vi "PC Streaming Host with slow - original.vi"() -> ()   [LabVIEW 2012]
uses:
  <vilib>/userdefined/High Color/nirio_resource_hc.ctl
  hv cluster control.ctl
  Slow cluster control.ctl
  <vilib>/FPGAPlugInAG/PXI-7951R/niLvFpga_Open_PXI-7951R.vi
  <vilib>/rvi/interface/common/dynamic/niFpgaDynamicAddResources.vi
  <vilib>/Utility/error.llb/Error Cluster From Error Code.vi
  <vilib>/rvi/errors/niLvFpgaAdjustHostInterfaceError.vi
  <vilib>/FPGAPlugInAG/Dynamic/niLvFpga_Close_Dynamic.vi
  <vilib>/rvi/interface/nirviOpenFPGA/nirviOpenFPGA.xnode
  FPGA Bitfiles/ModuDAQ_FPGATarget_TopLevelFPGAw8LE_8T5P+CgHwo4.lvbitx
  <vilib>/rvi/interface/nirviReadWriteControl/nirviReadWriteControl.xnode
  <vilib>/rvi/interface/nirviMethod/nirviMethod.xnode
  <vilib>/rvi/interface/nirviCloseFPGA/nirviCloseFPGA.xnode
  <vilib>/ptbypt/NI_PtbyPt.lvlib
  <vilib>/rvi/interface/Simulation/niFpgaSimulationCallBeginRW.vi
  CAENHVs/CAEN/labview/CAENHVWrapper/CAENHVWrapper.lvlib
  NiFpgaLv.dll
  <vilib>/FPGAPlugInAG/Dynamic/niLvFpga_ReadFifo_Dynamic.vi
  <vilib>/rvi/errors/niLvFpgaMergeErrorWithErrorCode.vi
panel:
  out "fast loop stop":bool
  in  "Channel Cluster":T1={"det_type"=["", "", "", "", "", "", "", ""], "Serial numbers"=["", "", "", "", "", "", "", ""], "Sources"=["", "", "", "", "", "", "", ""], "Trigger level"=[4000, 4000, 4000, 4000, 4000, 4000, 4000, 4000], "Data Record On/Off"=[FALSE, FALSE, FALSE, FALSE, FALSE, FALSE, FALSE, FALSE, TRUE, FALSE, FALSE, FALSE, FALSE, FALSE, FALSE, TRUE], "Number of Channels"=8}
  in  "HV Cluster":T2={"HV Power On/Off"=[TRUE, TRUE], "Set Voltage(V)"=["0", "0", "0", "0", "0", "0", "0", "0"], "HV Tolerance (%)"=1.0, "Current(uA)"=[]}
  out "created path":path
  out "File name":string
  out "Total Data Chunks to Write":dbl
  in  "Tab Control":T3(tab)
  in  "Write mode":bool
  out "directory exists - please wait":u8(slide)
  out "directory ok":bool
  in  "Write Enable":bool
  in  "File Path":path=path "G:/"
  out "File Writing Progress (%)":dbl(slide) scale=0.0..100.0
  in  "Slow Control On":bool
  in  "Fast Data On":bool
  in  "Number of Files to Write":u32=1
  in  "IP Address of NIST Time Server":string(combo)="ntp1.nikhef.nl"
  in  "VISA resource name":refnum<visa-resource-name>="COM8"
  out "HV Power On/Off":bool[](array[boolean])
  in  "HV Tolerance (%)":dbl=1.0
  out "HV(V)":sgl[](array[numeric])
  in  "IP adress HV2":string="1_0_0"
  in  "IP adress HV1":string="0_0_0"
  out "error HV":errorcluster
  out "Set Voltage":string[](array[string])=["0", "0", "0", "0", "0", "0", "0", "0"]
  out "Current(uA)":sgl[](array[numeric])
  in  "General Cluster":cluster{"Location":i16}={"Location"=1} {"Location" items=["Purdue", "NIKHEF", "Zurich", "???"]}
  in  "PXI address":T4="RIO0" caption="RIO Device"
  in  "det_type":string[](array[combo])=["NaI(Tl)", "NaI(Tl)", "NaI(Tl)", "NaI(Tl)", "NaI(Tl)", "NaI(Tl)", "NaI(Tl)", "NaI(Tl)"]
  in  "Serial numbers":string[](array[combo])=["SBJ593", "SBJ592", "SBJ590", "SBJ591", "SBJ588", "SBJ589", "SBJ586", "Other"]
  in  "Sources":string[](array[combo])=["Background", "Background", "Ti-44", "Ti-44", "Co-60", "Co-60", "Cs-137", "Cs-137"]
  in  "Trigger level":i16[](array[numeric])=[2000, 2000, 2000, 2000, 2000, 2000, 2000, 2000] caption="Trigger"
  in  "Data Record \nOn/Off":bool[](array[boolean])=[TRUE, TRUE, TRUE, TRUE, TRUE, TRUE, TRUE, TRUE]
  in  "Testpulse Cluster":T5={"Master Pulser On/Off"=FALSE, "Testpulse Turnaround Time (samples)"=14, "Pulse Separation (samples)"=0, "Pulse duration (samples)"=0}
  out "Samples per Data Chunk":u32
  in  "DAQ Info Cluster":T6={"Data Chunks per File"=1000, "Samples per Waveform"=95, "Pretrigger Samples"=15, "circular buffer length (samples)"=1000, "Waveforms per Data Chunk"=5000} {"Waveforms per Data Chunk" format="%.2p"}
  out "Average Throughput":dbl(graph)
  out "Loop Time":u32
  out "Inst. Throughput":dbl format="%#_6p"
  out "Elements in FIFO":u32(graph)
  out "FIFO Overflow":bool
  out "Current Chunk":u32
  out "Current File":i32
  out "Waveform Graph":dynamicdata(graph)
  out "Channel number displayed":i16=-1
  in  "Arduino read \nrate (Hz)":dbl=1.0
  out "Slow time":u64
  out "data":dbl[](array[numeric])
  in  "XON Character":u8=17 format="%.0x"
  in  "XOFF Character":u8=19 format="%.0x"
  out "Slow Cluster":T7
  out "read buffer":string
  out "Bad sensor?":string
  in  "Max Slow Entries per File":i32=86400
  out "Current Slow File":i32
  out "Current Slow Entry":i32
  out "Sensor out of bounds":bool
  out "Temperature":dbl(graph)
  out "Pressure":dbl(graph)
  out "magnetic field y coordinate":dbl(graph)
  out "total magnetic field":dbl(graph)
  out "magnetic field z coordinate":dbl(graph)
  out "magnetic field x coordinate":dbl(graph)
  out "humidity":dbl(graph)
  out "XML String":string
  out "Slow XML":string
  out "error out FAST":errorcluster
  out "error out SLOW":errorcluster
  out "error out XML":errorcluster
  out "NIST Time":u64
  out "NIST Time Failed to Read":bool
  in  "Minutes to wait":u32=5 min=3
  out "UTC format":bool=TRUE
  out "FPGA Timestamp":u64
  out "Time stamp string":string
  out "Stopped":bool
  in  "stop":bool
  # "Channel 0"
  # "Channel 1"
  # "Channel 2"
  # "Channel 3"
  # "Channel 4"
  # "Channel 5"
  # "Channel 6"
  # "Channel 7"
  # "Write continuously"
  # "Write finite number of files"
  # "Program will stop when number of Files to Write is Complete OR if stop is pressed."
  # "These parameters are set by the set_shutdown_HV vi!"
  # "Channel 0"
  # "Channel 1"
  # "Channel 2"
  # "Channel 3"
  # "Channel 4"
  # "Channel 5"
  # "Channel 6"
  # "Channel 7"
  # "This is not a cluster"
  # "Channel 0"
  # "Channel 1"
  # "Channel 2"
  # "Channel 3"
  # "Channel 4"
  # "Channel 5"
  # "Channel 6"
  # "Channel 7"
  # "TODO: Make this look like the \"detectors\" tab"
  # "Waveform/Data Chunk information"
  # "To compare directly on a scope: Horizontal scale: 200 ns/div Vertical scale: ~100 mV/div If 15 pretriggers, delay = 700 ns"
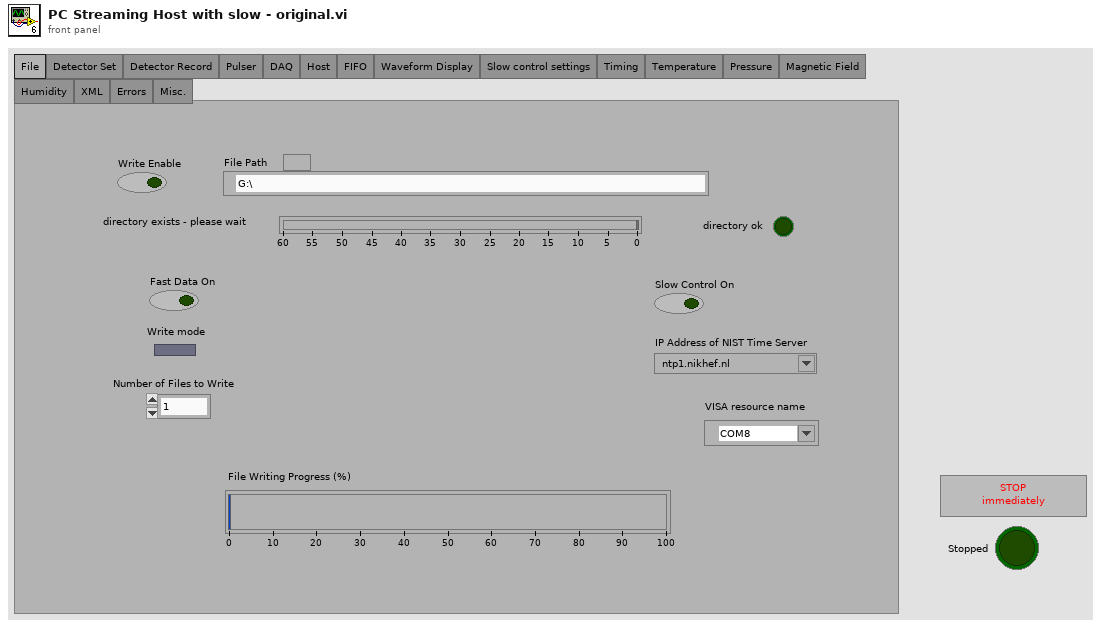
[diagram p1: front panel]
types:
  T1 = cluster{"det_type":string[], "Serial numbers":string[], "Sources":string[], "Trigger level":i16[], "Data Record On/Off":bool[], "Number of Channels":u8}
  T2 = typedef "hv cluster control.ctl" = cluster{"HV Power On/Off":bool[], "Set Voltage(V)":string[], "HV Tolerance (%)":dbl, "Current(uA)":dbl[]}
  T3 = enum32{"File", "Detector Set", "Detector Record", "Pulser", "DAQ", "Host", "FIFO", "Waveform Display", "Slow control settings", "Timing", "Temperature", "Pressure", "Magnetic Field", "Humidity", "XML", "Errors", "Misc."}
  T4 = typedef "nirio_resource_hc.ctl" = tag
  T5 = cluster{"Master Pulser On/Off":bool, "Testpulse Turnaround Time (samples)":u32, "Pulse Separation (samples)":u32, "Pulse duration (samples)":u32}
  T6 = cluster{"Data Chunks per File":u32, "Samples per Waveform":u32, "Pretrigger Samples":u32, "circular buffer length (samples)":u32, "Waveforms per Data Chunk":u32}
  T7 = typedef "Slow cluster control.ctl" = cluster{"Arduino \nParameters":dbl, "Total Number of \nSlow Parameters":i32, "UTC format?":bool, "Sensor Upper \nbounds":i32[], "Sensor Lower \nbounds":i32[], "Descriptions":string[], "datanames":string[]}
  T8 = enum16{"open", "replace", "create", "open or create", "replace or create", "replace or create with confirmation"}
  T9 = enum16{"big-endian, network order", "native, host order", "little-endian"}
  T10 = cluster{"Arduino Parameters":dbl, "Total Number of Slow Parameters":i32, "UTC format?":bool, "Sensor Upper bounds":i32[], "Sensor Lower bounds":i32[], "Descriptions":string[], "datanames":string[]}
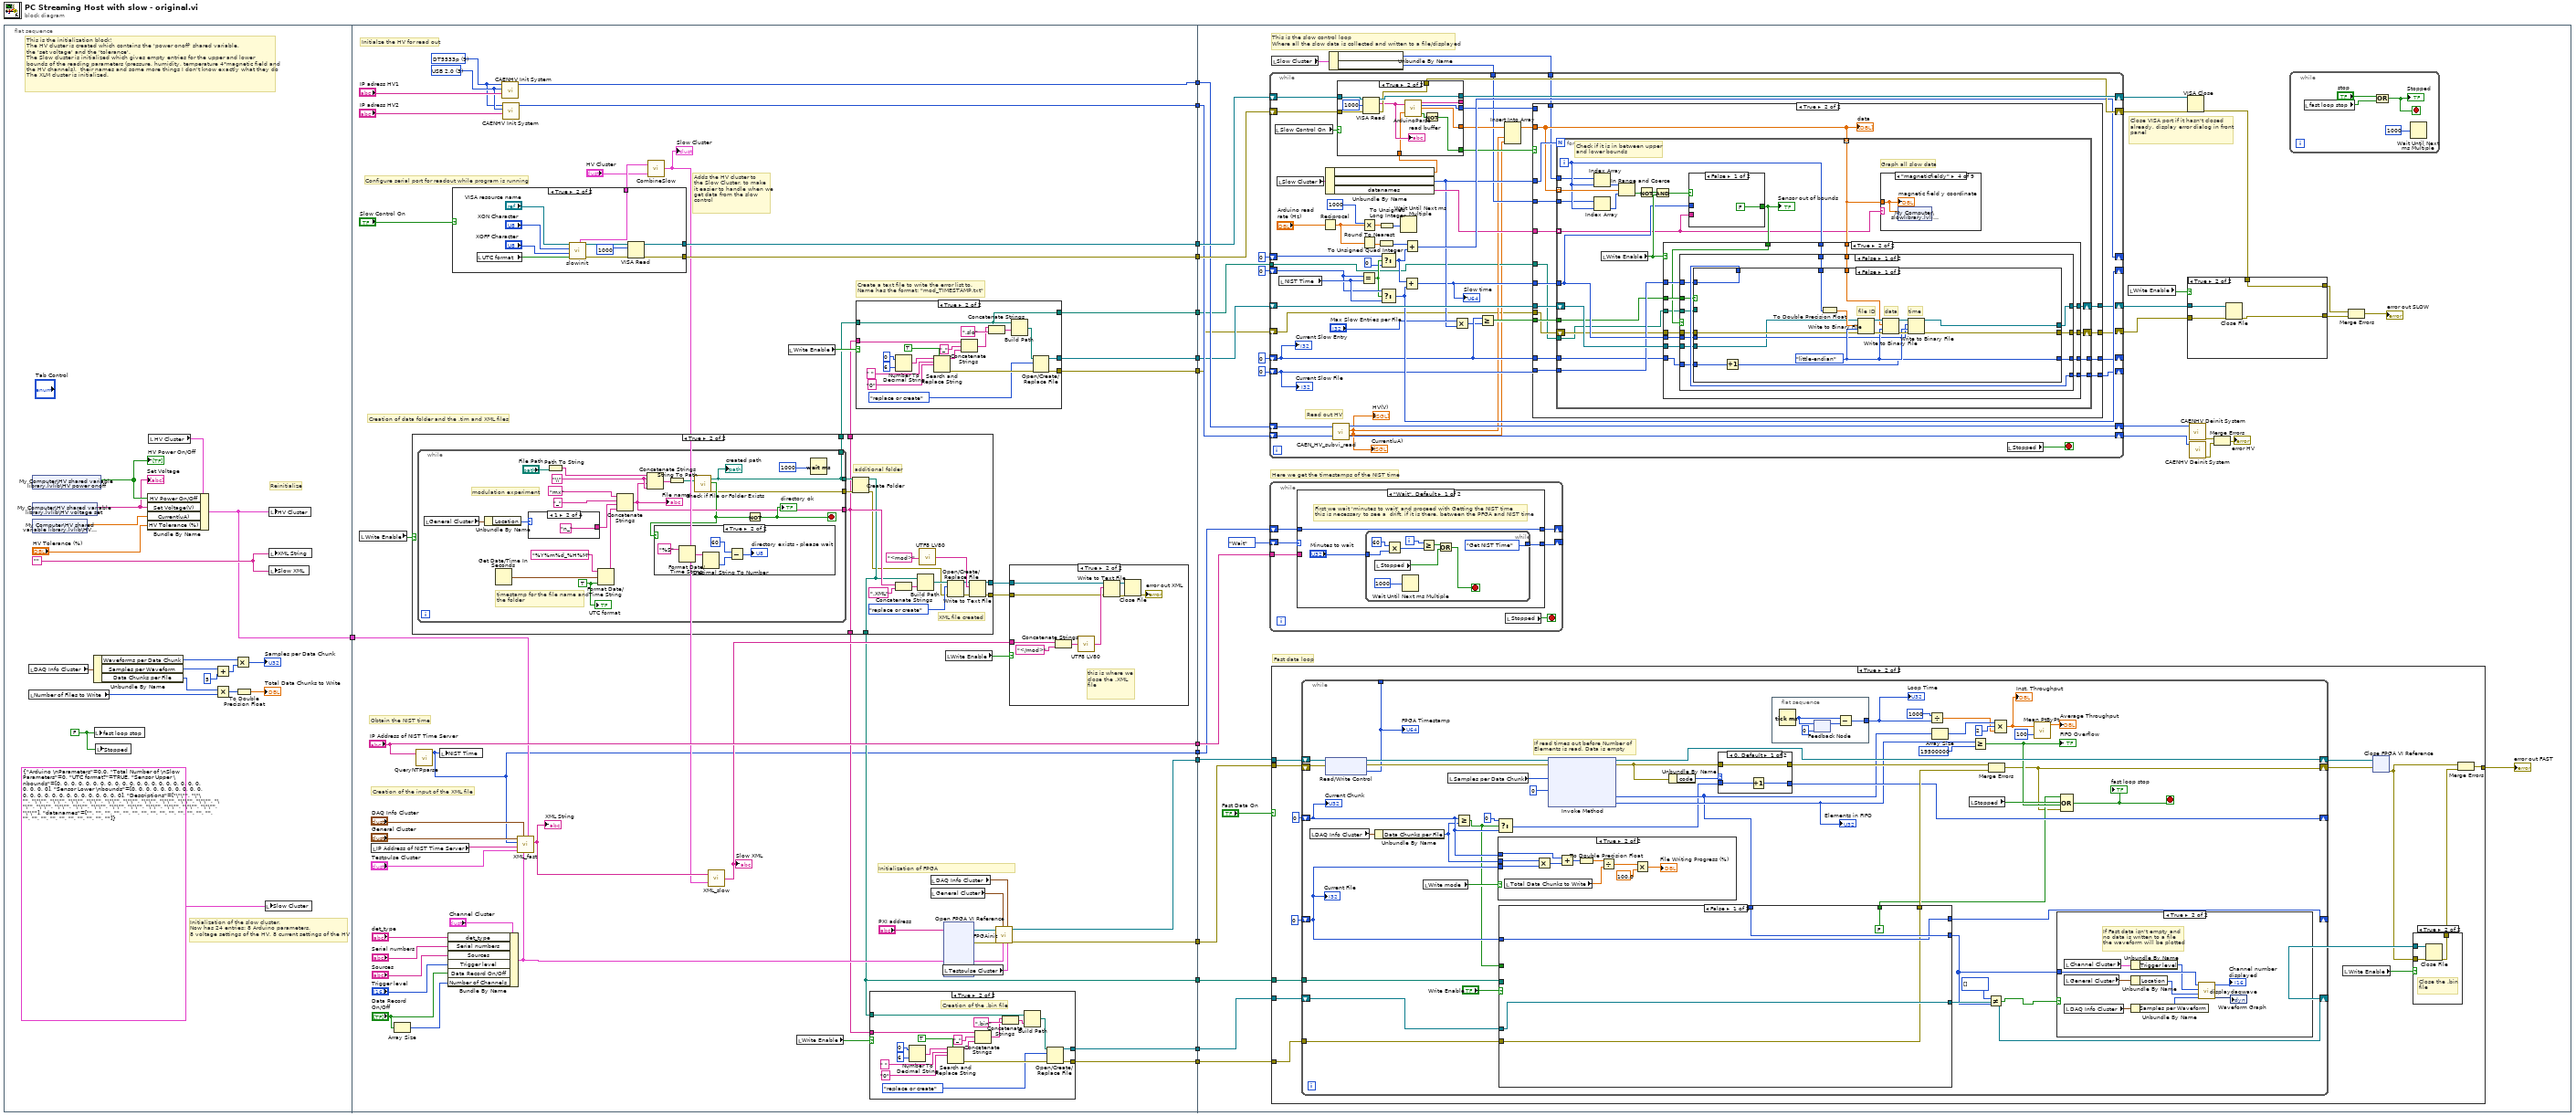
[diagram p0: block diagram]
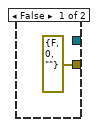
[diagram p2: hidden frame]
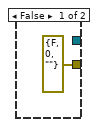
[diagram p3: hidden frame]
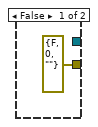
[diagram p6: hidden frame]
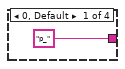
[diagram p7: hidden frame]
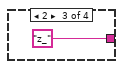
[diagram p8: hidden frame]
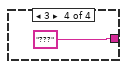
[diagram p9: hidden frame]
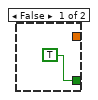
[diagram p11: hidden frame]
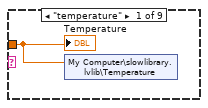
[diagram p13: hidden frame]
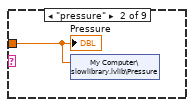
[diagram p14: hidden frame]
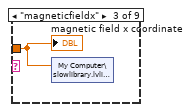
[diagram p15: hidden frame]
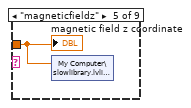
[diagram p16: hidden frame]
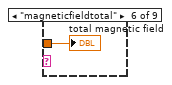
[diagram p17: hidden frame]
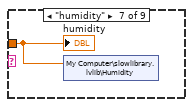
[diagram p18: hidden frame]
diagram:
  n1 = flat-sequence {
    tunnel: [w20] -> w4
    tunnel: ["IP Address of NIST Time Server"] -> w15
    tunnel: [w63] -> w14
    tunnel: [w62] -> w13
    tunnel: [w58] -> w12
    tunnel: [w57] -> w11
    tunnel: [w56] -> w10
    tunnel: [w47] -> w9
    tunnel: [w46] -> w8
    tunnel: [w45] -> w7
    tunnel: [w41] -> w6
    tunnel: [w40] -> w5
    tunnel: w4 -> [w39]
    tunnel: [w38] -> w3
    tunnel: [w37] -> w2
    tunnel: [w36] -> w1
    tunnel: w15 -> [w220]
    tunnel: w14 -> [w212]
    tunnel: w13 -> [w211]
    tunnel: w12 -> [w208]
    tunnel: w11 -> [w210]
    tunnel: w10 -> [w209]
    tunnel: w9 -> [w207]
    tunnel: w8 -> [w206]
    tunnel: w7 -> [w205]
    tunnel: w6 -> [w204]
    tunnel: w5 -> [w203]
    tunnel: w3 -> [w202]
    tunnel: w2 -> [w197]
    tunnel: w1 -> [w194]
    frame #0 {
      w17 = FALSE ("fast loop stop")
      w34 = ""
      # "Initialization of the slow cluster.\nNow has 24 entries: 8 Arduino parameters, \n8 voltage settings of the HV, 8 current settings of the HV"
      # "This is the initialization block!\nThe HV cluster is created which contains the 'power onoff' shared variable, \nthe 'set voltage' and the 'tolerance'.\nThe Slow cluster is initialized which gives empty entries for the upper and lower\nbounds of the reading parameters (pressure, humidity, temperature 4*magnetic field and\nthe HV channels),  their names and some more things I don't know exactly what they do\nThe XLM cluster is initialized."
      # "Reinitialize"
      n2 = local read "DAQ Info Cluster"() -> (w32:T6)
      n3 = local read "Number of Files to Write"() -> (w27:u32)
      n4 = shared-variable "My Computer\\HV shared variable library.lvlib\\HV power onoff"() -> (w22:bool[])  [unwired: 1 in, 1 out]
      "HV Power On/Off" <- w22
      n5 = shared-variable "My Computer\\HV shared variable library.lvlib\\HV voltage set"() -> (w21:string[])  [unwired: 1 in, 1 out]
      "Set Voltage" <- w21
      n6 = shared-variable "My Computer\\HV shared variable library.lvlib\\HV current"() -> (w18:dbl[])  [unwired: 1 in, 1 out]
      n7 = Unbundle By Name(w32) -> ("Waveforms per Data Chunk"=w24:u32, "Samples per Waveform"=w25:u32, "Data Chunks per File"=w26:u32)
      n8 = local write "fast loop stop"(w17) -> ()
      n9 = local write "Stopped"(w17) -> ()
      n10 = local read "HV Cluster"() -> (w33:T2)
      n11 = Bundle By Name(cluster=w33, "HV Power On/Off"=w22, "Set Voltage(V)"=w21, "Current(uA)"=w18, "HV Tolerance (%)"="HV Tolerance (%)") -> (w20:T2)
      n12 = Add(x=w25, y=u32 5) -> (x+y=w29:u32)
      n13 = Multiply(x=w26, y=w27) -> (x*y=w31:u32)
      n14 = Multiply(x=w24, y=w29) -> (x*y=→"Samples per Data Chunk":u32)
      n15 = To Double Precision Float(number=w31) -> (double precision float=→"Total Data Chunks to Write":dbl)
      n16 = local write "Slow Cluster"(T7 {"Arduino \nParameters"=0.0, "Total Number of \nSlow Parameters"=0, "UTC format?"=TRUE, "Sensor Upper \nbounds"=[0, 0, 0, 0, 0, 0, 0, 0, 0, 0, 0, 0, 0, 0, 0, 0, 0, 0, 0, 0, 0, 0, 0, 0], "Sensor Lower \nbounds"=[0, 0, 0, 0, 0, 0, 0, 0, 0, 0, 0, 0, 0, 0, 0, 0, 0, 0, 0, 0, 0, 0, 0, 0], "Descriptions"=["\"\"", "\"\"", "\"\"", "\"\"", "\"\"", "\"\"", "\"\"", "\"\"", "\"\"", "\"\"", "\"\"", "\"\"", "\"\"", "\"\"", "\"\"", "\"\"", "\"\"", "\"\"", "\"\"", "\"\"", "\"\"", "\"\"", "\"\"", "\"\""], "datanames"=["", "", "", "", "", "", "", "", "", "", "", "", "", "", "", "", "", "", "", "", "", "", "", ""]} ("Slow Cluster 2")) -> ()
      n17 = local write "HV Cluster"(w20) -> ()
      n18 = local write "XML String"(w34) -> ()
      n19 = local write "Slow XML"(w34) -> ()
    }
    frame #1 {
      w65 = 3 items=["TCP/IP"=0, "HS CAENET"=2, "USB 2.0"=3, "CONET Optical Link"=4, "USB VCP"=5] ("LinkType")
      w64 = u32 9 items=["SY1527", "SY2527", "SY4527", "SY5527", "N568", "V65XX", "N1470", "V8100", "", "DT5533p"] ("system")
      # "Obtain the NIST time"
      # "Adds the HV cluster to\nthe Slow Cluster, to make\nit easier to handle when we\nget data from the slow\ncontrol"
      # "Initialization of FPGA"
      # "Initialze the HV for read out"
      # "Create a text file to write the error list to.  \nName has the format: \"mod_TIMESTAMP.txt\""
      # "Creation of the input of the XML file"
      # "Configure serial port for readout while program is running"
      # "Creation of data folder and the .tim and XML files"
      n20 = local read "Write Enable"() -> (w86:bool)
      n21 = local read "IP Address of NIST Time Server"() -> (w77:string)
      n22 = Array Size(array="Data Record \nOn/Off") -> (size(s)=w75:i32)
      n23 = case shown="True" w86 {
        tunnel: [_ w158] -> w59
        tunnel: [_ w150] -> w61
        tunnel: [_ w148] -> w48
        tunnel: [_ w148] -> w42
        tunnel: [_ w147] -> w41
        tunnel: [errorcluster {"status"=FALSE, "code"=0, "source"=""} ("error out") w145] -> w35
        frame False {
        }
        frame True {
          # "XML file created"
          # "additional folder"
          n24 = while {
            tunnel: [w161] -> w159
            tunnel: [w163] -> w160
            tunnel: [w163] -> w158
            tunnel: [w168] -> w148
            stop <- w173 stop-if-true
            w169 = "\\" ("string")
            w176 = TRUE ("UTC format")
            # "modulation experiment"
            # "timestamp for the file name and the folder"
            n25 = local read "General Cluster"() -> (w166:cluster{"Location":i16})
            n26 = Unbundle By Name(w166) -> ("Location"=w165:i16)
            n27 = Get Date/Time In Seconds() -> (seconds since 1Jan1904=w177:timestamp)
            n28 = case shown="1" w165 {
              tunnel: ["p_" ("string") "n_" ("string") "z_" ("string") "???"] -> w167
              frame 0, Default {
              }
              frame 1 {
              }
              frame 2 {
              }
              frame 3 {
              }
            }
            n29 = Path To String(path="File Path") -> (string=w179:string)
            n30 = Format Date/Time String(time format string (%c)="%Y%m%d_%H%M", seconds (now)=w177, UTC format=w176) -> (date/time string=w170:string)
            n31 = Concatenate Strings("mx" ("string"), "_" ("string"), w167, w170) -> (w168:string)
            "File name" <- w168
            n32 = Concatenate Strings(w179, w169, w168, w169) -> (w180:string)
            n33 = String To Path(string=w180) -> (path=w164:path)
            n34 = call <vilib>:"Check if File or Folder Exists.vi"("path"=w164) -> ("error out"=w161:errorcluster, "file or folder exists?"=w162:bool, "dup path"=w163:path)  [unwired: 8 in]
            "created path" <- w163
            n35 = case shown="True" w162 {
              frame False {
              }
              frame True {
                n36 = Format Date/Time String(time format string (%c)="%S") -> (date/time string=w188:string)  [unwired: 2 in]
                n37 = Decimal String To Number(string=w188) -> (number=w186:i32)  [unwired: 2 in, 1 out]
                n38 = Subtract(x=60, y=w186) -> (x-y=→"directory exists - please wait":i32)
              }
            }
            n39 = Not(x=w162) -> (.not. x?=w173:bool)
            "directory ok" <- w173
            n40 = Wait (ms)(milliseconds to wait=1000) -> ()  [unwired: 1 out]
            "UTC format" <- w176
          }
          n41 = Create Folder(path (use dialog)=w160, error in=w159) -> (created path=w147:path, error out=w146:errorcluster)  [unwired: 1 in, 1 out]
          n42 = Concatenate Strings(w148, ".XML" ("substring (\"\")")) -> (w154:string)
          n43 = Build Path(base path=w147, name or relative path=w154) -> (appended path=w153:path)
          n44 = call "UTF8 LV80.vi"("text"="<mod>") -> ("utf-8 text out"=w157:string)
          n45 = Open/Create/Replace File(file path (use dialog)=w153, error in=w146, operation (0:open)=T8."replace or create") -> (refnum out=w156:refnum<file>, error out=w155:errorcluster)  [unwired: 3 in, 1 out]
          n46 = Write to Text File(file (use dialog)=w156, text=w157, error in=w155) -> (refnum out=w150:refnum<file>, error out=w145:errorcluster)  [unwired: 1 in, 1 out]
        }
      }
      n47 = call "QueryNTPparse.vi"("IP Address of NIST Server"="IP Address of NIST Time Server") -> ("NTP Time (server time)"=w38:u64)  [unwired: 1 in, 2 out]
      n48 = local write "NIST Time"(w38) -> ()
      n49 = Bundle By Name(cluster="Channel Cluster", "det_type"="det_type", "Serial numbers"="Serial numbers", "Sources"="Sources", "Trigger level"="Trigger level", "Data Record On/Off"="Data Record \nOn/Off", "Number of Channels"=w75) -> (w44:T1)
      n50 = case shown="True" "Slow Control On" {
        tunnel: [_ w143] -> w63
        tunnel: [_ w142] -> w62
        tunnel: [_ w134] -> w85
        frame False {
        }
        frame True {
          n51 = local read "UTC format"() -> (w137:bool)
          n52 = call "slowinit.vi"("UTC format"=w137, "XOFF Character"="XOFF Character", "XON Character"="XON Character", "VISA resource name"="VISA resource name") -> ("error IO"=w135:errorcluster, "VISA resource name out"=w136:refnum<visa-resource-name>, "Slow Cluster"=w134:T10)  [unwired: 5 in]
          n53 = VISA Read(VISA resource name=w136, byte count=u32 1000, error in (no error)=w135) -> (VISA resource name out=w143:refnum<visa-resource-name>, error out=w142:errorcluster)  [unwired: 2 out]
        }
      }
      n54 = call "CAENHV Init System.vi"("Arg"="IP adress HV1", "LinkType"=w65, "system"=w64) -> ("handle"=w57:i32)  [unwired: 7 in, 1 out]
      n55 = call "CAENHV Init System.vi"("Arg"="IP adress HV2", "LinkType"=w65, "system"=w64) -> ("handle"=w56:i32)  [unwired: 7 in, 1 out]
      n56 = call "XML_fast.vi"("HV Cluster"=w39, "Channel \nCluster"=w44, "DAQ Info Cluster"="DAQ Info Cluster", "Testpulse \nCluster"="Testpulse Cluster", "IP Address of NIST Time Server"=w77, "NIST Time"=w38, "General Cluster"="General Cluster") -> ("XML String"=w80:string)  [unwired: 4 in]
      "XML String" <- w80
      n57 = call "CombineSlow.vi"("HV Cluster"="HV Cluster", "Slow Cluster in"=w85) -> ("Slow Cluster"=w43:T7)
      "Slow Cluster" <- w43
      n58 = call "XML_slow.vi"("Slow Cluster"=w43, "Input String"=w80) -> ("Output String"=w81:string)
      "Slow XML" <- w81
      n59 = local read "Write Enable"() -> (w60:bool)
      n60 = local read "Write Enable"() -> (w49:bool)
      n61 = case shown="True" w60 {
        tunnel: [_ w117] -> w58
        tunnel: w48 -> [_ w109]
        tunnel: w59 -> [_ w108]
        tunnel: [_ w108] -> w40
        tunnel: [errorcluster {"status"=FALSE, "code"=0, "source"=""} ("error out") w107] -> w37
        frame False {
        }
        frame True {
          n62 = Number To Decimal String(number=0, width (-)=i16 6) -> (decimal integer string=w124:string)
          n63 = Search and Replace String(replace all?=TRUE ("replace all? (F)"), input string=w124, search string=" ", replace string="0" ("replace string (\"\")")) -> (result string=w114:string, error out=w119:errorcluster)  [unwired: 4 in, 2 out]
          n64 = Concatenate Strings(w109, "_" ("string"), w114) -> (w112:string)
          n65 = Concatenate Strings(w112, ".slo" ("substring (\"\")")) -> (w116:string)
          n66 = Build Path(base path=w108, name or relative path=w116) -> (appended path=w120:path)
          n67 = Open/Create/Replace File(file path (use dialog)=w120, error in=w119, operation (0:open)=T8."replace or create") -> (refnum out=w117:refnum<file>, error out=w107:errorcluster)  [unwired: 3 in, 1 out]
        }
      }
      n68 = case shown="True" w49 {
        tunnel: [_ w98] -> w47
        tunnel: w42 -> [_ w90]
        tunnel: w41 -> [_ w89]
        tunnel: [errorcluster {"status"=FALSE, "code"=0, "source"=""} ("error out") w88] -> w36
        frame False {
        }
        frame True {
          # "Creation of the .bin file"
          n69 = Number To Decimal String(number=0, width (-)=i16 6) -> (decimal integer string=w105:string)
          n70 = Search and Replace String(replace all?=TRUE ("replace all? (F)"), input string=w105, search string=" ", replace string="0" ("replace string (\"\")")) -> (result string=w95:string, error out=w100:errorcluster)  [unwired: 4 in, 2 out]
          n71 = Concatenate Strings(w90, "_" ("string"), w95) -> (w93:string)
          n72 = Concatenate Strings(w93, ".bin" ("substring (\"\")")) -> (w97:string)
          n73 = Build Path(base path=w89, name or relative path=w97) -> (appended path=w101:path)
          n74 = Open/Create/Replace File(file path (use dialog)=w101, error in=w100, operation (0:open)=T8."replace or create") -> (refnum out=w98:refnum<file>, error out=w88:errorcluster)  [unwired: 3 in, 1 out]
        }
      }
      n75 = local read "DAQ Info Cluster"() -> (w53:T6)
      n76 = local read "General Cluster"() -> (w52:cluster{"Location":i16})
      n77 = local read "Testpulse Cluster"() -> (w51:T5)
      n78 = xnode "Open FPGA VI Reference"("resource name"="PXI address") -> ("FPGA VI Reference Out"=w55:refnum<k20>, "error out"=w54:errorcluster)  [unwired: 1 in]
      n79 = local read "Write Enable"() -> (w68:bool)
      n80 = call "FPGAinit.vi"("Testpulse Cluster"=w51, "DAQ Info Cluster"=w53, "Channel Cluster"=w44, "General Cluster"=w52, "error in"=w54, "FPGA VI Reference In"=w55) -> ("error out"=w45:errorcluster, "FPGA VI Reference Out"=w46:refnum<k20>)  [unwired: 4 in]
      n81 = case shown="True" w68 {
        tunnel: w61 -> [_ w133]
        tunnel: w81 -> [_ w128]
        tunnel: w35 -> [_ w127]
        frame False {
        }
        frame True {
          # "this is where we close the .XML file"
          n82 = Concatenate Strings(w128, "</mod>" ("string")) -> (w129:string)
          n83 = call "UTF8 LV80.vi"("text"=w129) -> ("utf-8 text out"=w132:string)
          n84 = Write to Text File(file (use dialog)=w133, text=w132, error in=w127) -> (refnum out=w131:refnum<file>, error out=w126:errorcluster)  [unwired: 1 in, 1 out]
          n85 = Close File(refnum=w131, error in=w126) -> (error out=→"error out XML":errorcluster)  [unwired: 1 out]
        }
      }
    }
    frame #2 {
      # "This is the slow control loop\nWhere all the slow data is collected and written to a file/displayed"
      # "Fast data loop"
      # "Close VISA port if it hasn't closed already, display error dialog in front panel"
      # "Here we get the timestamps of the NIST time"
      n86 = while {
        shift-right: [w613] -> _
        shift-left: enum16{"Wait", "Get NIST Time", "Write"}."Wait" -> [w614]
        shift-right: [w612] -> _
        shift-left: w202 -> [w611]
        tunnel: w220 -> [w610]
        stop <- w609 stop-if-true
        n87 = case shown="\"Wait\", Default" w614 {
          tunnel: [w617 enum16{"Wait", "Get NIST Time", "Write"}."Wait"] -> w613
          tunnel: [w616 w633] -> w612
          tunnel: w611 -> [w616 w630]
          tunnel: w610 -> [_ w629]
          frame "Wait", Default {
            # "First we wait 'minutes to wait' and proceed with Getting the NIST time\nthis is necessary to see a  drift, if it is there, between the PFGA and NIST time"
            n88 = while {
              tunnel: [enum16{"Wait", "Get NIST Time", "Write"}."Get NIST Time"] -> w617
              tunnel: "Minutes to wait" -> [w619]
              i -> [w622]
              stop <- w623 stop-if-true
              n89 = local read "Stopped"() -> (w621:bool)
              n90 = Multiply(x=60, y=w619) -> (x*y=w618:u32)
              n91 = Wait Until Next ms Multiple(millisecond multiple=u32 1000 ("y")) -> ()  [unwired: 1 out]
              n92 = Greater Or Equal?(x=w622, y=w618) -> (x >= y?=w624:bool)
              n93 = Or(x=w624, y=w621) -> (x .or. y?=w623:bool)
            }
          }
          frame "Get NIST Time" {
            # "Here we get the NIST time"
            n94 = call "QueryNTPparse.vi"("IP Address of NIST Server"=w629) -> ("NTP Time (server time)"=w632:u64, "Time stamp string"=→"Time stamp string":string)  [unwired: 1 in, 1 out]
            "NIST Time" <- w632
            n95 = Equal?(x=w630, y=w632) -> (x = y?=w631:bool)
            "NIST Time Failed to Read" <- w631
            n96 = Select(t=w630, s=w631, f=w632) -> (s? t:f=w633:u64)
          }
        }
        n97 = local read "Stopped"() -> (w609:bool)
      }
      n98 = local read "Slow Cluster"() -> (w224:T7)
      n99 = case shown="True" "Fast Data On" {
        tunnel: w207 -> [_ w449]
        tunnel: w206 -> [_ w448]
        tunnel: w205 -> [w439 w447]
        tunnel: w204 -> [_ w446]
        tunnel: [w439 w441] -> w195
        tunnel: w194 -> [_ w440]
        frame False {
        }
        frame True {
          n100 = while {
            shift-right: [w460] -> w444
            shift-left: w447 -> [w479]
            shift-right: [w486] -> _
            shift-left: u32 0 -> [w483]
            shift-right: [w471] -> _
            shift-left: 0 ("number") -> [w472]
            shift-right: [w487] -> w451
            shift-left: w449 -> [w488]
            tunnel: [w476] -> _
            tunnel: w446 -> [w464]
            shift-right: [w503] -> w445
            shift-left: w448 -> [w466]
            tunnel: w440 -> [w459]
            stop <- w473 stop-if-true
            # "If read times out before Number of Elements is read, Data is empty"
            n101 = local read "DAQ Info Cluster"() -> (w468:T6)
            n102 = xnode "Read/Write Control"("FPGA VI Reference In"=w466, "error in"=w479) -> ("FPGA VI Reference Out"=w478:refnum<k20>, "error out"=w477:errorcluster, "Timestamp"=w476:u64)
            "FPGA Timestamp" <- w476
            n103 = Unbundle By Name(w468) -> ("Data Chunks per File"=w467:u32)
            n104 = local read "Write mode"() -> (w480:bool)
            n105 = local read "Samples per Data Chunk"() -> (w465:u32)
            n106 = Greater Or Equal?(x=w483, y=w467) -> (x >= y?=w461:bool)
            n107 = Select(t=u32 0, s=w461, f=w483) -> (s? t:f=w463:u32)
            n108 = case shown="True" w480 {
              tunnel: w472 -> [_ w522]
              tunnel: w483 -> [_ w520]
              tunnel: w467 -> [_ w513]
              frame False {
              }
              frame True {
                n109 = local read "Total Data Chunks to Write"() -> (w517:dbl)
                n110 = Multiply(x=w513, y=w522) -> (x*y=w521:u32)
                n111 = Add(x=w520, y=w521) -> (x+y=w519:u32)
                n112 = To Double Precision Float(number=w519) -> (double precision float=w518:dbl)
                n113 = Divide(x=w518, y=w517) -> (x/y=w515:dbl)
                n114 = Multiply(x=w515, y=100.0) -> (x*y=→"File Writing Progress (%)":dbl)
              }
            }
            n115 = xnode "Invoke Method"("FPGA VI Reference In"=w478, "error in"=w477, "Number of Elements"=w465, "Timeout (ms)"=0) -> ("FPGA VI Reference Out"=w503:refnum<k20>, "error out"=w500:errorcluster, "Data"=w481:i16[], "Elements Remaining"=w482:u32)
            "Elements in FIFO" <- w482
            n116 = case shown="False" "Write Enable" {
              tunnel: w481 -> [w530 w532]
              tunnel: [w530 _] -> w470
              tunnel: w461 -> [_ w541]
              tunnel: [w527 w540] -> w489
              tunnel: [w531 w539] -> w487
              tunnel: w488 -> [w531 w538]
              tunnel: w472 -> [w529 w537]
              tunnel: [w529 w536] -> w471
              tunnel: [FALSE w535] -> w462
              tunnel: w464 -> [_ w534]
              tunnel: w459 -> [w527 w533]
              frame False {
              }
              frame True {
                n117 = case shown="False" w541 {
                  tunnel: w532 -> [w546 w574]
                  tunnel: [w545 w576] -> w540
                  tunnel: w538 -> [w550 w589]
                  tunnel: [w549 w582] -> w539
                  tunnel: w537 -> [w544 w562]
                  tunnel: [w544 w561] -> w536
                  tunnel: [FALSE w560] -> w535
                  tunnel: w534 -> [_ w563]
                  tunnel: w533 -> [w542 w559]
                  frame False {
                    # "binary writing will write 0 if there is no data"
                    n118 = Not Equal?(x=w546, y=i16[] []) -> (x != y?=w547:bool)
                    n119 = case shown="True" w547 {
                      tunnel: w550 -> [w552 w558]
                      tunnel: [w552 w557] -> w549
                      tunnel: [w551 w556] -> w545
                      tunnel: w546 -> [_ w554]
                      tunnel: w542 -> [w551 w553]
                      frame False {
                      }
                      frame True {
                        n120 = Write to Binary File(file (use dialog)=w558, data=w554, error in=w553, 9:T9."little-endian" ("byte order (0:big-endian, network order)")) -> (refnum out=w557:refnum<file>, error out=w556:errorcluster)  [unwired: 2 in, 1 out]
                      }
                    }
                  }
                  frame True {
                    # "little-endian is windows and linux way of writing and reading binary not the standard in labview !?!"
                    # "opening the new ones"
                    # "closing files"
                    n121 = Increment(x=w562) -> (x+1=w561:i32)
                    n122 = Number To Decimal String(number=w561, width (-)=i16 6) -> (decimal integer string=w591:string)
                    n123 = Close File(refnum=w589, error in=w559) -> (error out=w588:errorcluster)  [unwired: 1 out]
                    n124 = local read "File name"() -> (w570:string)
                    n125 = Search and Replace String(replace all?=TRUE ("replace all? (F)"), input string=w591, search string=" ", replace string="0" ("replace string (\"\")"), error in=w588) -> (result string=w581:string, error out=w587:errorcluster)  [unwired: 3 in, 2 out]
                    n126 = Concatenate Strings(w570, "_" ("string"), w581) -> (w577:string)
                    n127 = local read "Samples per Data Chunk"() -> (w569:u32)
                    n128 = Concatenate Strings(w577, ".bin" ("substring (\"\")")) -> (w579:string)
                    n129 = Equal?(x="Write mode", y=TRUE) -> (x = y?=w568:bool)
                    n130 = Equal?(x="Number of Files to Write", y=w561) -> (x = y?=w567:bool)
                    n131 = And(x=w567, y=w568) -> (x .and. y?=w560:bool)
                    n132 = Build Path(base path=w563, name or relative path=w579) -> (appended path=w586:path)
                    n133 = Open/Create/Replace File(file path (use dialog)=w586, error in=w587, operation (0:open)=T8."replace or create") -> (refnum out=w583:refnum<file>, error out=w584:errorcluster)  [unwired: 3 in, 1 out]
                    n134 = Array Size(array=w574) -> (size(s)=w573:i32)
                    n135 = Equal?(x=w573, y=w569) -> (x = y?=w572:bool)
                    n136 = Not Equal?(x=w574, y=i16[] []) -> (x != y?=w575:bool)
                    n137 = And(x=w575, y=w572) -> (x .and. y?=w571:bool)
                    n138 = case shown="True" w571 {
                      tunnel: w584 -> [w596 w603]
                      tunnel: w583 -> [w597 w602]
                      tunnel: [w597 w601] -> w582
                      tunnel: [w596 w600] -> w576
                      tunnel: w574 -> [_ w599]
                      frame False {
                      }
                      frame True {
                        n139 = Write to Binary File(file (use dialog)=w602, data=w599, error in=w603, 9:T9."little-endian" ("byte order (0:big-endian, network order)")) -> (refnum out=w601:refnum<file>, error out=w600:errorcluster)  [unwired: 2 in, 1 out]
                      }
                    }
                  }
                }
              }
            }
            n140 = Unbundle By Name(w500) -> ("code"=w501:i32)
            n141 = case shown="0, Default" w501 {
              tunnel: [w606 errorcluster {"status"=FALSE, "code"=0, "source"=""} ("error constant")] -> w490
              tunnel: w500 -> [w606 _]
              tunnel: w463 -> [w605 w607]
              tunnel: [w604 w607] -> w486
              frame 0, Default {
                n142 = Increment(x=w605) -> (x+1=w604:u32)
              }
              frame -50400 {
                # "Timeout"
              }
            }
            n143 = flat-sequence {
              tunnel: [w526] -> w494
              frame #0 {
                n144 = Tick Count (ms)() -> (millisecond timer value=w525:u32)
                n145 = feedback #1(u32 0 ("millisecond timer value")) -> (w524:u32)
                n146 = feedback-in #1(w525) -> ()
                n147 = Subtract(x=w525, y=w524) -> (x-y=w526:u32)
              }
            }
            n148 = Divide(x=u32 1000, y=w494) -> (x/y=w496:dbl)
            n149 = Array Size(array=w481) -> (size(s)=w499:i32)
            n150 = local read "Stopped"() -> (w475:bool)
            n151 = Greater Or Equal?(x=w482, y=u32 19500000) -> (x >= y?=w474:bool)
            "FIFO Overflow" <- w474
            n152 = Not Equal?(x=i16[] [], y=w470) -> (x != y?=w458:bool)
            n153 = Merge Errors(w490, w489) -> (w460:errorcluster)
            n154 = Compound Arithmetic op=MULTIPLY(w499, 2 ("y"), w496) -> (w493:dbl)
            "Inst. Throughput" <- w493
            n155 = call <vilib>:"Mean PtByPt.vi"("x"=w493, "sample length"=100) -> ("mean"=→"Average Throughput":dbl)  [unwired: 2 in, 1 out]
            n156 = case shown="True" w458 {
              tunnel: w470 -> [_ w512]
              frame False {
              }
              frame True {
                # "If Fast data isn't empty and\nno data is written to a file\nthe waveform will be plotted"
                n157 = local read "Channel Cluster"() -> (w510:T1)
                n158 = local read "General Cluster"() -> (w508:cluster{"Location":i16})
                n159 = local read "DAQ Info Cluster"() -> (w506:T6)
                n160 = Unbundle By Name(w510) -> ("Trigger level"=w509:i16[])
                n161 = Unbundle By Name(w508) -> ("Location"=w507:i16)
                n162 = Unbundle By Name(w506) -> ("Samples per Waveform"=w505:u32)
                n163 = call "displaydaqwave.vi"("Samples per Waveform"=w505, "Location"=w507, "Trigger level"=w509, "Waveform from DAQ"=w512) -> ("Waveform Graph"=→"Waveform Graph":dynamicdata, "Channel number displayed"=→"Channel number displayed":i16)  [unwired: 6 in]
              }
            }
            n164 = Compound Arithmetic op=OR(w462, w475, w474, w460) -> (w473:bool)
            "fast loop stop" <- w473
            "Loop Time" <- w494
            "Current Chunk" <- w483
            "Current File" <- w472
          }
          n165 = local read "Write Enable"() -> (w453:bool)
          n166 = xnode "Close FPGA VI Reference"("FPGA VI Reference In"=w445, "error in"=w444) -> ("error out"=w443:errorcluster)
          n167 = case shown="True" w453 {
            tunnel: w443 -> [w454 w456]
            tunnel: w451 -> [_ w457]
            tunnel: [w454 w455] -> w442
            frame False {
            }
            frame True {
              # "Close the .bin\nfile"
              n168 = Close File(refnum=w457, error in=w456) -> (error out=w455:errorcluster)  [unwired: 1 out]
            }
          }
          n169 = Merge Errors(w443, w442) -> (w441:errorcluster)
        }
      }
      "error out FAST" <- w195
      n170 = Unbundle By Name(w224) -> ("Sensor Upper \nbounds"=w214:i32[], "Sensor Lower \nbounds"=w213:i32[])
      n171 = while {
        shift-right: [w269] -> _
        shift-left: u64 0 -> [w273]
        shift-right: [w266] -> _
        shift-left: u64 0 -> [w271]
        shift-right: [w252] -> w219
        shift-left: w208 -> [w275]
        shift-right: [w248] -> _
        shift-left: 0 -> [w249]
        shift-right: [w247] -> _
        shift-left: 0 -> [w251]
        tunnel: w214 -> [w241]
        tunnel: w213 -> [w240]
        tunnel: w203 -> [w231]
        shift-right: [w277] -> w216
        shift-left: w212 -> [w239]
        shift-right: [w276] -> w215
        shift-left: w211 -> [w238]
        shift-right: [w235] -> w218
        shift-left: w210 -> [w237]
        shift-right: [w233] -> w217
        shift-left: w209 -> [w236]
        shift-right: [w228] -> w196
        shift-left: w197 -> [w229]
        stop <- w232 stop-if-true
        # "Read out HV"
        n172 = local read "Slow Control On"() -> (w255:bool)
        n173 = local read "Slow Cluster"() -> (w260:T7)
        n174 = local read "NIST Time"() -> (w274:u64)
        n175 = Reciprocal(x="Arduino read \nrate (Hz)") -> (1/x=w263:dbl)
        n176 = Unbundle By Name(w260) -> ("Arduino \nParameters"=w256:dbl, "Total Number of \nSlow Parameters"=w245:i32, "datanames"=w253:string[])
        n177 = call "CAEN_HV_subvi_read.vi"("handle HV1"=w237, "handle HV2"=w236) -> ("handle HV1 out"=w235:i32, "HV"=w234:sgl[], "Current"=w230:sgl[], "handle HV2 out"=w233:i32)  [unwired: 1 in, 1 out]
        "HV(V)" <- w234
        "Current(uA)" <- w230
        n178 = case shown="True" w255 {
          tunnel: [_ w289] -> w277
          tunnel: [_ w288] -> w276
          tunnel: [_ w286] -> w259
          tunnel: [_ w285] -> _
          tunnel: [TRUE w281] -> w254
          tunnel: [_ w283] -> w258
          tunnel: w256 -> [_ w282]
          tunnel: w239 -> [_ w280]
          tunnel: w238 -> [_ w279]
          frame False {
          }
          frame True {
            n179 = VISA Read(VISA resource name=w280, byte count=u32 1000, error in (no error)=w279) -> (VISA resource name out=w289:refnum<visa-resource-name>, read buffer=w287:string, error out=w288:errorcluster)  [unwired: 1 out]
            "read buffer" <- w287
            n180 = call "ArduinoParse.vi"("read buffer"=w287, "Expected Arduino Parameters"=w282) -> ("Number Arduino Parameters"=w286:i32, "Arduino Data Names"=w285:string[], "Arduino Data"=w283:dbl[], "Arduino Read Failed?"=w284:bool)
            n181 = Not(x=w284) -> (.not. x?=w281:bool)
          }
        }
        n182 = Equal?(x=w273, y=w274) -> (x = y?=w272:bool)
        n183 = Multiply(x=u32 1000 ("millisecond multiple"), y=w263) -> (x*y=w265:dbl)
        n184 = Round To Nearest(number=w263) -> (nearest integer value=w262:dbl)
        n185 = To Unsigned Quad Integer(1:w262) -> (0:w261:u64)
        n186 = To Unsigned Long Integer(number=w265) -> (unsigned 32bit integer=w264:u32)
        n187 = Select(t=w271, s=w272, f=0) -> (s? t:f=w267:u64)
        n188 = Select(t=w273, s=w272, f=w274) -> (s? t:f=w269:u64)
        n189 = Wait Until Next ms Multiple(millisecond multiple=w264) -> ()  [unwired: 1 out]
        n190 = Add(x=w267, y=w269) -> (x+y=w242:u64)
        "Slow time" <- w242
        n191 = Add(x=w261, y=w267) -> (x+y=w266:u64)
        n192 = Multiply(x="Max Slow Entries per File", y=w245) -> (x*y=w244:i32)
        n193 = Greater Or Equal?(x=w249, y=w244) -> (x >= y?=w250:bool)
        n194 = Insert Into Array(array=w258, new element #1=w234, new element #2=w230) -> (w257:dbl[])  [unwired: 1 in]
        n195 = case shown="True" w254 {
          tunnel: w275 -> [w294 w310]
          tunnel: w242 -> [_ w309]
          tunnel: [w294 w306] -> w252
          tunnel: w259 -> [_ _]
          tunnel: w257 -> [_ w300]
          tunnel: w253 -> [_ w308]
          tunnel: w245 -> [_ w307]
          tunnel: w251 -> [w292 w305]
          tunnel: w250 -> [_ w304]
          tunnel: w249 -> [w293 w303]
          tunnel: [w293 w302] -> w248
          tunnel: [w292 w301] -> w247
          tunnel: w241 -> [_ w299]
          tunnel: w240 -> [_ w298]
          tunnel: w231 -> [_ w295]
          tunnel: w229 -> [w291 w297]
          tunnel: [w291 w296] -> w228
          frame False {
          }
          frame True {
            n196 = for {
              N: w307 -> [_]
              tunnel: w309 -> [w330]
              tunnel: w300 -> [w333] mode=indexing
              tunnel: w308 -> [w318] mode=indexing
              tunnel: w300 -> [w319] mode=indexing
              tunnel: w305 -> [w327]
              tunnel: w304 -> [w325]
              tunnel: w303 -> [w324]
              tunnel: [w323] -> w302
              tunnel: [w322] -> w301
              shift-right: [w328] -> w306
              shift-left: w310 -> [w329]
              tunnel: w299 -> [w317]
              tunnel: w298 -> [w316]
              shift-right: [w313] -> w296
              shift-left: w297 -> [w312]
              tunnel: w295 -> [w311]
              i -> [w326]
              # "Check if it is in between upper \nand lower bounds"
              # "Graph all slow data"
              n197 = Index Array(array=w317, index=w326) -> (element=w314:i32)
              n198 = Index Array(array=w316, index=w326) -> (element=w315:i32)
              n199 = local read "Write Enable"() -> (w331:bool)
              n200 = In Range and Coerce(upper limit=w314, x=w333, lower limit=w315) -> (In Range?=w321:bool)  [unwired: 1 out]
              n201 = Not(x=w321) -> (.not. x?=w334:bool)
              n202 = And(x=w334, y=w331) -> (x .and. y?=w332:bool)
              n203 = case shown="False" w332 {
                tunnel: w318 -> [_ w427]
                tunnel: w330 -> [_ _]
                tunnel: [FALSE ("Sensor out of bounds") TRUE ("Sensor out of bounds")] -> w320
                frame False {
                }
                frame True {
                  "Bad sensor?" <- w427
                }
              }
              "Sensor out of bounds" <- w320
              n204 = case shown="True" w331 {
                tunnel: [w343 w359] -> w322
                tunnel: w319 -> [_ w358]
                tunnel: w330 -> [_ w357]
                tunnel: w329 -> [w345 w356]
                tunnel: [w345 w355] -> w328
                tunnel: w327 -> [w343 w354]
                tunnel: w326 -> [_ w353]
                tunnel: w325 -> [_ w352]
                tunnel: w324 -> [w344 w351]
                tunnel: [w344 w350] -> w323
                tunnel: w320 -> [_ w349]
                tunnel: w311 -> [_ w348]
                tunnel: [w342 w347] -> w313
                tunnel: w312 -> [w342 w346]
                frame False {
                }
                frame True {
                  n205 = case shown="False" w349 {
                    tunnel: [w372 w424] -> w359
                    tunnel: w358 -> [w371 _]
                    tunnel: w357 -> [w370 _]
                    tunnel: w356 -> [w369 w423]
                    tunnel: [w368 w423] -> w355
                    tunnel: w354 -> [w367 w424]
                    tunnel: w353 -> [w366 _]
                    tunnel: w352 -> [w365 _]
                    tunnel: w351 -> [w364 w425]
                    tunnel: [w363 w425] -> w350
                    tunnel: w348 -> [w362 _]
                    tunnel: [w361 w422] -> w347
                    tunnel: w346 -> [w360 w422]
                    frame False {
                      n206 = case shown="False" w365 {
                        tunnel: [w380 w394] -> w372
                        tunnel: w371 -> [w382 w402]
                        tunnel: w370 -> [w381 w401]
                        tunnel: w369 -> [w374 w400]
                        tunnel: [w376 w398] -> w368
                        tunnel: w367 -> [w380 w397]
                        tunnel: w366 -> [w379 w396]
                        tunnel: w364 -> [w378 _]
                        tunnel: [w377 0] -> w363
                        tunnel: w362 -> [_ w392]
                        tunnel: [w373 w390] -> w361
                        tunnel: w360 -> [w375 w391]
                        frame False {
                          w383 = T9."little-endian" ("byte order (0:big-endian, network order)")
                          # "time"
                          # "data"
                          # "file ID"
                          n207 = Increment(x=w378) -> (x+1=w377:i32)
                          n208 = To Double Precision Float(number=w379) -> (double precision float=w384:dbl)
                          n209 = Write to Binary File(file (use dialog)=w374, data=w384, error in=w375, 9:w383) -> (refnum out=w387:refnum<file>, error out=w388:errorcluster)  [unwired: 2 in, 1 out]
                          n210 = Write to Binary File(file (use dialog)=w387, data=w382, error in=w388, 9:w383) -> (refnum out=w386:refnum<file>, error out=w385:errorcluster)  [unwired: 2 in, 1 out]
                          n211 = Write to Binary File(file (use dialog)=w386, data=w381, error in=w385, 9:w383) -> (refnum out=w376:refnum<file>, error out=w373:errorcluster)  [unwired: 2 in, 1 out]
                        }
                        frame True {
                          w403 = T9."little-endian" ("byte order (0:big-endian, network order)")
                          w393 = TRUE ("replace all? (F)")
                          # "time"
                          # "data"
                          # "file ID"
                          # "opening the new ones"
                          # "closing files"
                          n212 = Increment(x=w397) -> (x+1=w394:i32)
                          n213 = Number To Decimal String(number=w394, width (-)=i16 6) -> (decimal integer string=w418:string)
                          n214 = Close File(refnum=w400, error in=w391) -> (error out=w416:errorcluster)  [unwired: 1 out]
                          n215 = local read "File name"() -> (w409:string)
                          n216 = Search and Replace String(replace all?=w393, case sensitive?=w393, input string=w418, search string=" ", replace string="0" ("replace string (\"\")"), error in=w416) -> (result string=w413:string, error out=w415:errorcluster)  [unwired: 2 in, 2 out]
                          n217 = Concatenate Strings(w409, "_" ("string"), w413) -> (w410:string)
                          n218 = Concatenate Strings(w410, ".slo" ("substring (\"\")")) -> (w411:string)
                          n219 = Build Path(base path=w392, name or relative path=w411) -> (appended path=w389:path)
                          n220 = Open/Create/Replace File(file path (use dialog)=w389, error in=w415, operation (0:open)=T8."replace or create") -> (refnum out=w399:refnum<file>)  [unwired: 3 in, 2 out]
                          n221 = To Double Precision Float(number=w396) -> (double precision float=w404:dbl)
                          n222 = Write to Binary File(file (use dialog)=w399, data=w404, 9:w403) -> (refnum out=w407:refnum<file>, error out=w408:errorcluster)  [unwired: 3 in, 1 out]
                          n223 = Write to Binary File(file (use dialog)=w407, data=w402, error in=w408, 9:w403) -> (refnum out=w406:refnum<file>, error out=w405:errorcluster)  [unwired: 2 in, 1 out]
                          n224 = Write to Binary File(file (use dialog)=w406, data=w401, error in=w405, 9:w403) -> (refnum out=w398:refnum<file>, error out=w390:errorcluster)  [unwired: 2 in, 1 out]
                        }
                      }
                    }
                    frame True {
                    }
                  }
                }
              }
              n225 = case shown="\"magneticfieldy\"" w318 {
                tunnel: w319 -> [w335 w336 w337 w338 w339 w340 w341 _ _]
                frame "temperature" {
                  n226 = shared-variable "My Computer\\slowlibrary.lvlib\\Temperature"(w335) -> ()  [unwired: 1 in, 1 out]
                  "Temperature" <- w335
                }
                frame "pressure" {
                  n227 = shared-variable "My Computer\\slowlibrary.lvlib\\Pressure"(w336) -> ()  [unwired: 1 in, 1 out]
                  "Pressure" <- w336
                }
                frame "magneticfieldx" {
                  n228 = shared-variable "My Computer\\slowlibrary.lvlib\\B_x"(w337) -> ()  [unwired: 1 in, 1 out]
                  "magnetic field x coordinate" <- w337
                }
                frame "magneticfieldy" {
                  n229 = shared-variable "My Computer\\slowlibrary.lvlib\\B_y"(w338) -> ()  [unwired: 1 in, 1 out]
                  "magnetic field y coordinate" <- w338
                }
                frame "magneticfieldz" {
                  n230 = shared-variable "My Computer\\slowlibrary.lvlib\\B_z"(w339) -> ()  [unwired: 1 in, 1 out]
                  "magnetic field z coordinate" <- w339
                }
                frame "magneticfieldtotal" {
                  "total magnetic field" <- w340
                }
                frame "humidity" {
                  n231 = shared-variable "My Computer\\slowlibrary.lvlib\\Humidity"(w341) -> ()  [unwired: 1 in, 1 out]
                  "humidity" <- w341
                }
                frame "seconds" {
                }
                frame "", Default {
                }
              }
            }
            "data" <- w300
          }
        }
        n232 = local read "Stopped"() -> (w232:bool)
        "Current Slow Entry" <- w249
        "Current Slow File" <- w251
      }
      n233 = local read "Write Enable"() -> (w225:bool)
      n234 = VISA Close(VISA resource name=w216, error in (no error)=w215) -> (error out=w193:errorcluster)
      n235 = case shown="True" w225 {
        tunnel: w219 -> [_ w434]
        tunnel: w196 -> [w429 w433]
        tunnel: w193 -> [w430 w431]
        tunnel: [w429 w432] -> w192
        tunnel: [w430 w431] -> w191
        frame False {
        }
        frame True {
          n236 = Close File(refnum=w434, error in=w433) -> (error out=w432:errorcluster)  [unwired: 1 out]
        }
      }
      n237 = call "CAENHV Deinit System.vi"("handle"=w218) -> ("error out"=w223:errorcluster)  [unwired: 10 in]
      n238 = call "CAENHV Deinit System.vi"("handle"=w217) -> ("error out"=w222:errorcluster)  [unwired: 10 in]
      n239 = Merge Errors(w223, w222) -> (→"error HV":errorcluster)
      n240 = while {
        stop <- w436 stop-if-true
        n241 = local read "fast loop stop"() -> (w435:bool)
        n242 = Compound Arithmetic op=OR("stop", w435) -> (w436:bool)
        "Stopped" <- w436
        n243 = Wait Until Next ms Multiple(millisecond multiple=u32 1000 ("y")) -> ()  [unwired: 1 out]
      }
      n244 = Merge Errors(w191, w192) -> (→"error out SLOW":errorcluster)
    }
  }
